vi "Generate File Header.vi"(8 "error in (no error)":errorcluster, 11 "LUnit Test Vector in":refnum<class "LUnit Test Vector.lvclass">) -> (0 "error out":errorcluster, 2 "Header":string, 3 "LUnit Test Vector out":refnum<class "LUnit Test Vector.lvclass">)   [LabVIEW 2020, in "LUnit Test Vector.lvclass"]
uses:
  LUnit Test Vector.lvclass
  LUnit Test Vector.lvclass/LUnit Test Vector.ctl
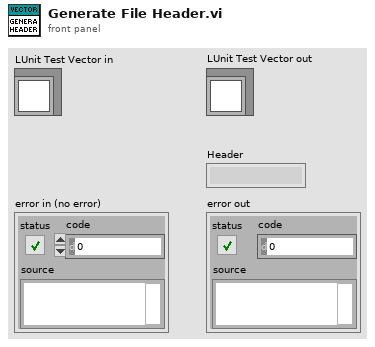
[diagram p1: front panel]
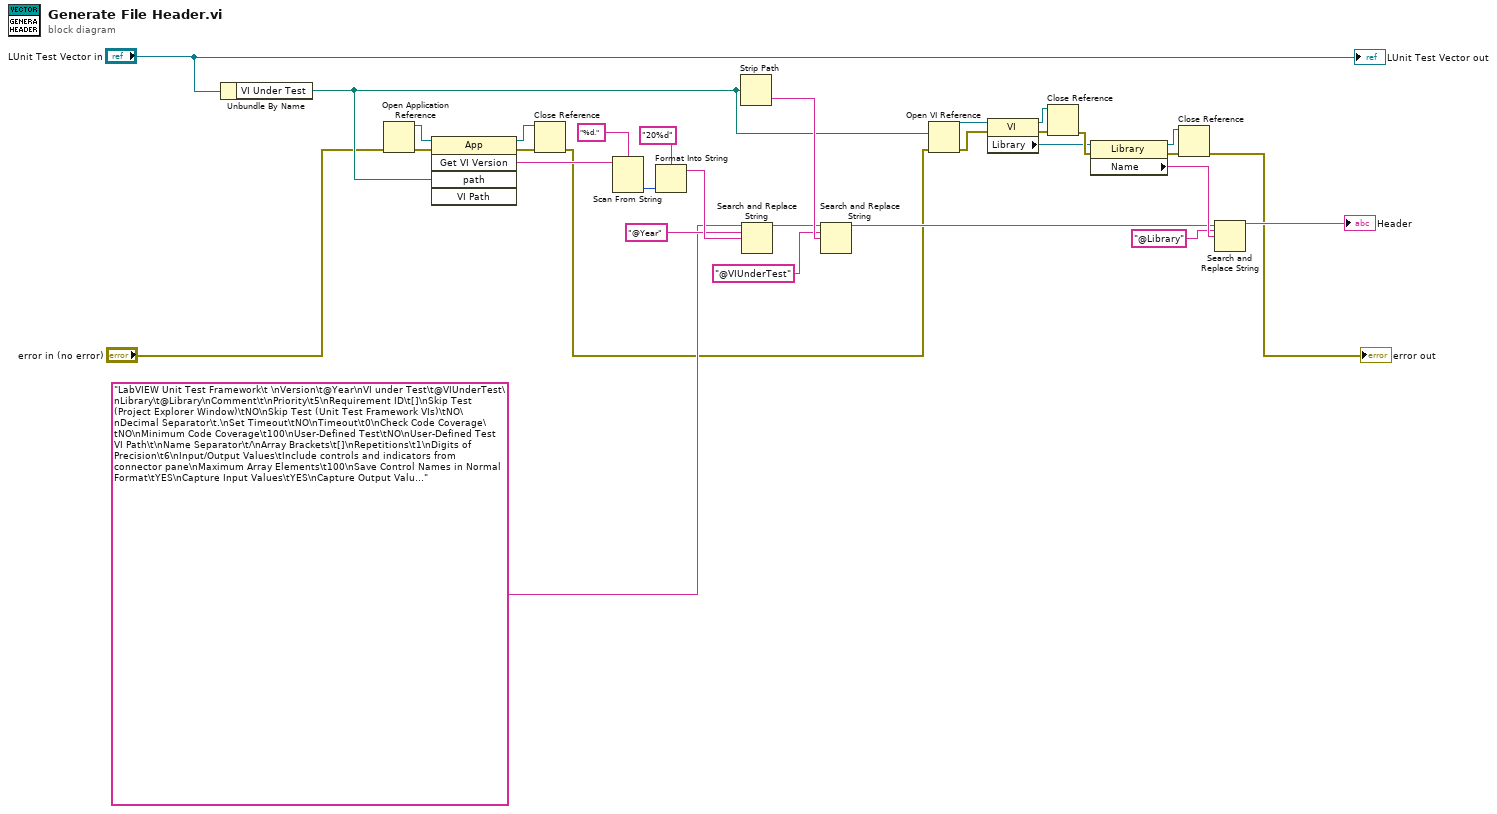
[diagram p0: block diagram]
diagram:
  n1 = Unbundle By Name("LUnit Test Vector in") -> ("VI Under Test"=w3:path)
  n2 = Open Application Reference(8:"error in (no error)") -> (0:w7:errorcluster, 3:w8:refnum<vi>)  [unwired: 3 in]
  n3 = invoke class="App" method="Get VI Version"(reference=w8, error in=w7, "path"=w3) -> (reference out=w5:refnum<vi>, error out=w6:errorcluster, "GetVIVers"=w4:string)  [unwired: 2 in, 2 out]
  n4 = Close Reference(reference=w5, error in (no error)=w6) -> (error out=w1:errorcluster)
  n5 = Scan From String(format string="%d.", input string=w4) -> (output 1=w12:i32)  [unwired: 3 in, 3 out]
  n6 = Format Into String(format string="20%d", w12) -> (resulting string=w16:string)  [unwired: 2 in, 1 out]
  n7 = Strip Path(path=w3) -> (name=w19:string)  [unwired: 1 out]
  n8 = Search and Replace String(input string="LabVIEW Unit Test Framework\t \nVersion\t@Year\nVI under Test\t@VIUnderTest\nLibrary\t@Library\nComment\t\nPriority\t5\nRequirement ID\t[]\nSkip Test (Project Explorer Window)\tNO\nSkip Test (Unit Test Framework VIs)\tNO\nDecimal Separator\t.\nSet Timeout\tNO\nTimeout\t0\nCheck Code Coverage\tNO\nMinimum Code Coverage\t100\nUser-Defined Test\tNO\nUser-Defined Test VI Path\t\nName Separator\t/\nArray Brackets\t[]\nRepetitions\t1\nDigits of Precision\t6\nInput/Output Values\tInclude controls and indicators from connector pane\nMaximum Array Elements\t100\nSave Control Names in Normal Format\tYES\nCapture Input Values\tYES\nCapture Output Values\tYES\nSet Automatic Error Handling\tAs is\nRemove Breakpoints\tYES\n", search string="@Year", replace string=w16) -> (result string=w18:string)  [unwired: 5 in, 3 out]
  n9 = Search and Replace String(input string=w18, search string="@VIUnderTest", replace string=w19) -> (result string=w27:string)  [unwired: 5 in, 3 out]
  n10 = Open VI Reference(vi path=w3, error in (no error)=w1) -> (vi reference=w9:refnum<vi>, error out=w25:errorcluster)  [unwired: 4 in]
  n11 = property class="VI"(reference=w9, error in=w25) -> (reference out=w22:refnum<vi>, error out=w21:errorcluster, "Library"=w20:refnum<vi>)
  n12 = Close Reference(reference=w22, error in (no error)=w21) -> (error out=w26:errorcluster)
  n13 = property class="Library"(reference=w20, error in=w26) -> (reference out=w24:refnum<vi>, error out=w23:errorcluster, "Name"=w29:string)
  n14 = Close Reference(reference=w24, error in (no error)=w23) -> (error out=→"error out":errorcluster)
  n15 = Search and Replace String(input string=w27, search string="@Library", replace string=w29) -> (result string=→"Header":string)  [unwired: 5 in, 3 out]
  "LUnit Test Vector out" <- "LUnit Test Vector in"
